vi "Load Database.vi"(7 "Box ID Array":u8[](array[numeric])=[1], 8 "error in (no error)":errorcluster, 10 "Calibration Mode":bool=TRUE, 11 "Battery Simulator 1200 Driver in":refnum<class "BS120x.lvclass">) -> (0 "error out":errorcluster, 1 "Specific Frames":refnum<k21>[](array[refnum]), 2 "XNET Database":refnum<k21>, 3 "Battery Simulator 1200 Driver out":refnum<class "BS120x.lvclass">)   [LabVIEW 2021, in "BS120x Driver.lvlib" / "BS120x.lvclass"]
uses:
  BS120x.lvclass
  BS120x.lvclass/BS120x.ctl
  <resource>/objmgr/xnet.rc
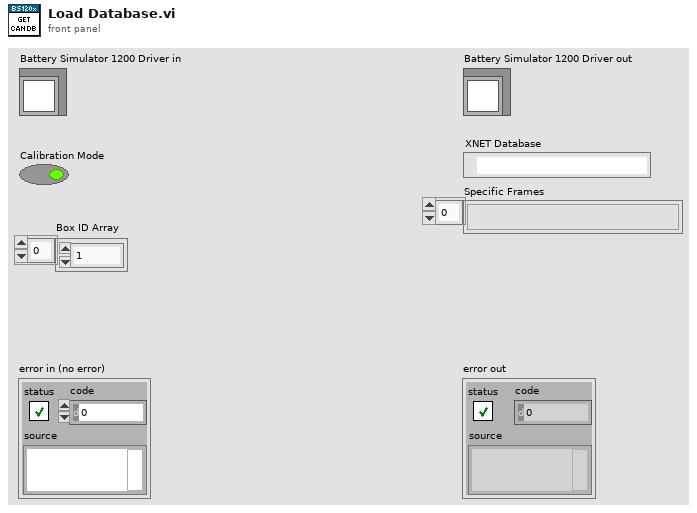
[diagram p1: front panel]
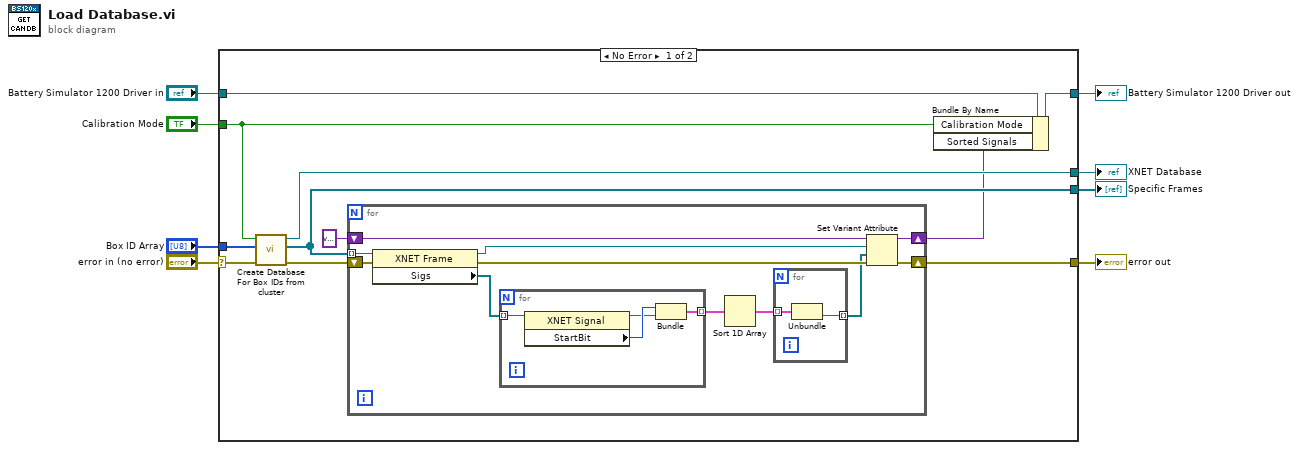
[diagram p0: block diagram]
diagram:
  n1 = case shown="No Error" "error in (no error)" {
    selector: "error in (no error)" -> [w19 w38]
    tunnel: [w12 w38] -> w7
    tunnel: [w16 w37] -> w5
    tunnel: "Battery Simulator 1200 Driver in" -> [w17 w37]
    tunnel: "Calibration Mode" -> [w18 _]
    tunnel: "Box ID Array" -> [w15 _]
    tunnel: [w11 _] -> w2
    tunnel: [w14 _] -> w1
    frame No Error {
      n2 = call "Create Database For Box IDs from cluster.vi"("error in (no error)"=w19, "Box ID Array"=w15, "Calibration mode"=w18) -> ("error out"=w13:errorcluster, "Specific Frames"=w11:refnum<k21>[], "XNET Database out"=w14:refnum<k21>)  [unwired: 6 in]
      n3 = for {
        tunnel: w11 -> [w26] mode=indexing
        shift-right: [w22] -> w12
        shift-left: w13 -> [w27]
        shift-right: [w24] -> w9
        shift-left: variant -> [w25]
        n4 = property class="XNET Frame"(reference=w26, error in=w27) -> (reference out=w20:refnum<k21>, error out=w23:errorcluster, "Sigs"=w30:refnum<k21>[])
        n5 = for {
          tunnel: w30 -> [w35] mode=indexing
          tunnel: [w33] -> w29 mode=indexing
          n6 = property class="XNET Signal"(reference=w35) -> (reference out=w34:refnum<k21>, "StartBit"=w36:u32)  [unwired: 1 in, 1 out]
          n7 = Bundle("StartBit"=w36, w34) -> (w33:cluster{"StartBit":u32, refnum<k21>})  [unwired: 1 in]
        }
        n8 = Sort 1D Array(array=w29) -> (sorted array=w28:cluster{"StartBit":u32, refnum<k21>}[])
        n9 = for {
          tunnel: w28 -> [w32] mode=indexing
          tunnel: [w31] -> w21 mode=indexing
          n10 = Unbundle(w32) -> (w31:refnum<k21>)  [unwired: 1 out]
        }
        n11 = Set Variant Attribute(Variant=w25, name=w20, value=w21, error in=w23) -> (Variant out=w24:variant, error out=w22:errorcluster)  [unwired: 1 out]
      }
      n12 = Bundle By Name(cluster=w17, "Calibration Mode"=w18, "Sorted Signals"=w9) -> (w16:refnum<class "BS120x.lvclass">)
    }
    frame Error {
    }
  }
  "error out" <- w7
  "Battery Simulator 1200 Driver out" <- w5
  "XNET Database" <- w1
  "Specific Frames" <- w2
